vi "StimFile (G3)-Create.vi"(0 "File":T1, 7 "Npts":i32=-1, 11 "error in (no error)":errorcluster) -> (4 "File out":T1, 8 "Y":dbl[](array[numeric]), 15 "error out":errorcluster)   [LabVIEW 2020]
uses:
  Waveform VIs/File VIs/StimFile-Params.ctl
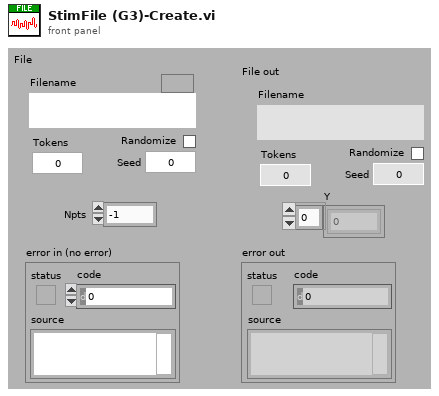
[diagram p1: front panel]
types:
  T1 = typedef "StimFile-Params.ctl" = cluster{"Filename":path, "Signal":dbl[], "Channel":i32, "stream":bool, "offset":i32, "nreps":i32, "loops":i32, "Randomize":bool, "order":i32[], "Seed":i32, "Tokens":i32}
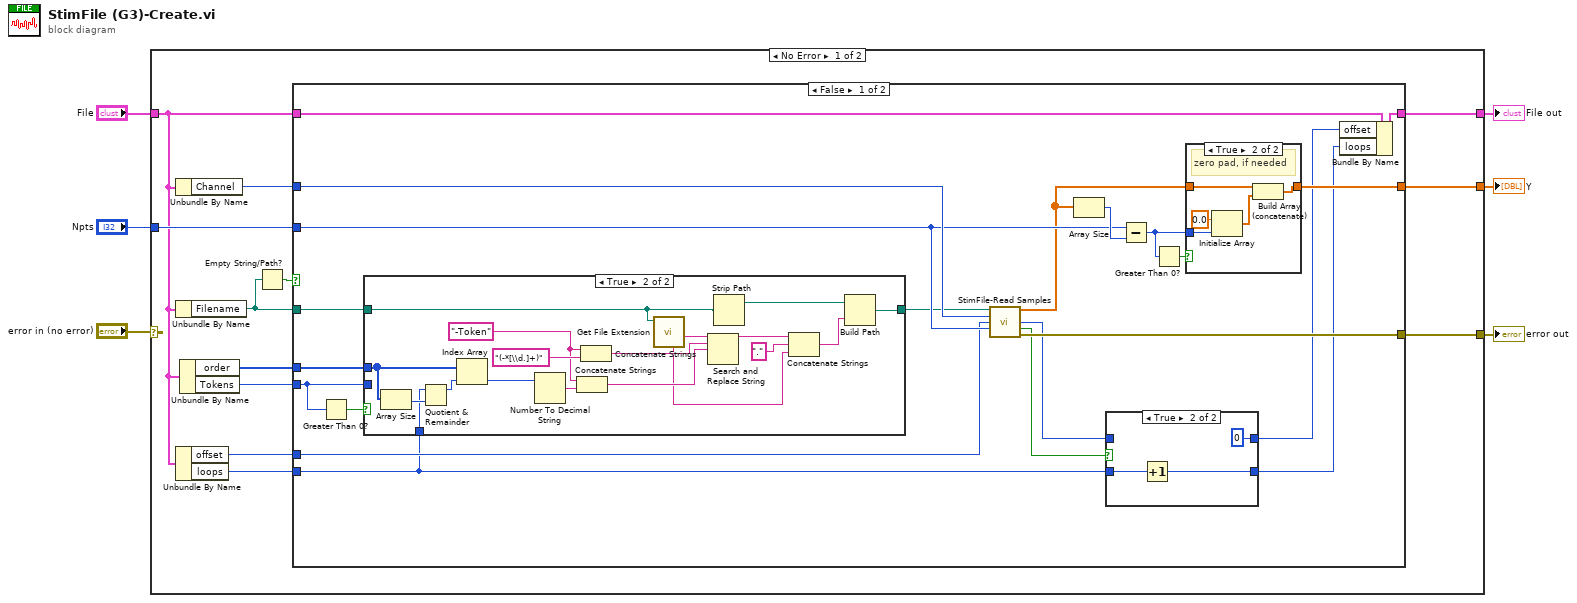
[diagram p0: block diagram]
diagram:
  n1 = case shown="No Error" "error in (no error)" {
    selector: "error in (no error)" -> [_ w71]
    tunnel: "File" -> [w9 _]
    tunnel: "Npts" -> [w17 _]
    tunnel: [w18 w71] -> w3
    tunnel: [w12 _] -> w2
    tunnel: [w11 _] -> w1
    frame No Error {
      n2 = Unbundle By Name(w9) -> ("Channel"=w14:i32)
      n3 = Unbundle By Name(w9) -> ("Filename"=w15:path)
      n4 = Unbundle By Name(w9) -> ("offset"=w13:i32, "loops"=w10:i32)
      n5 = Unbundle By Name(w9) -> ("order"=w7:i32[], "Tokens"=w8:i32)
      n6 = Empty String/Path?(string/path=w15) -> (empty?=w16:bool)
      n7 = case shown="False" w16 {
        tunnel: w15 -> [w24 _]
        tunnel: [w39 _] -> w18
        tunnel: w17 -> [w31 _]
        tunnel: w14 -> [w32 _]
        tunnel: w13 -> [w25 _]
        tunnel: w9 -> [w35 w70]
        tunnel: [w34 w70] -> w12
        tunnel: [w33 _] -> w11
        tunnel: w10 -> [w19 _]
        tunnel: w8 -> [w22 _]
        tunnel: w7 -> [w20 _]
        frame False {
          n8 = Greater Than 0?(x=w22) -> (x > 0?=w23:bool)
          n9 = case shown="True" w23 {
            tunnel: w24 -> [w40 w50]
            tunnel: w22 -> [_ _]
            tunnel: [w40 w48] -> w21
            tunnel: w20 -> [_ w44]
            tunnel: w19 -> [_ w42]
            frame False {
            }
            frame True {
              w57 = "-Token"
              n10 = Array Size(array=w44) -> (size(s)=w43:i32)
              n11 = Quotient & Remainder(x=w42, y=w43) -> (x-y*floor(x/y)=w41:i32)  [unwired: 1 out]
              n12 = Index Array(array=w44, index=w41) -> (element=w56:i32)
              n13 = Number To Decimal String(number=w56) -> (decimal integer string=w55:string)  [unwired: 1 in]
              n14 = Concatenate Strings(w57, w55) -> (w52:string)
              n15 = Concatenate Strings(w57, "(-*[\\d.]+)" ("string")) -> (w53:string)
              n16 = call <vilib>:"Get File Extension.vi"("file"=w50) -> ("filename without extension"=w54:string, "unmodified file extension"=w45:string)  [unwired: 6 in, 3 out]
              n17 = Search and Replace String(input string=w54, search string=w53, replace string=w52) -> (result string=w47:string)  [unwired: 5 in, 3 out]
              n18 = Strip Path(path=w50) -> (stripped path=w49:path)  [unwired: 1 out]
              n19 = Concatenate Strings(w47, "." ("string"), w45) -> (w51:string)
              n20 = Build Path(base path=w49, name or relative path=w51) -> (appended path=w48:path)
            }
          }
          n21 = call "StimFile-Read Samples.vi"("Filename"=w21, "channel"=w32, "offset in"=w25, "Npts"=w31) -> ("Samples"=w30:dbl[], "offset out"=w28:i32, "end of file?"=w29:bool, "error out"=w39:errorcluster)  [unwired: 8 in]
          n22 = Array Size(array=w30) -> (size(s)=w38:i32)
          n23 = case shown="True" w29 {
            tunnel: w19 -> [w60 w62]
            tunnel: w28 -> [w59 _]
            tunnel: [w59 0] -> w27
            tunnel: [w60 w61] -> w26
            frame False {
            }
            frame True {
              n24 = Increment(x=w62) -> (x+1=w61:i32)
            }
          }
          n25 = Subtract(x=w31, y=w38) -> (x-y=w36:i32)
          n26 = Greater Than 0?(x=w36) -> (x > 0?=w37:bool)
          n27 = case shown="True" w37 {
            tunnel: w30 -> [w64 w69]
            tunnel: w36 -> [_ w66]
            tunnel: [w64 w68] -> w33
            frame False {
            }
            frame True {
              # "zero pad, if needed"
              n28 = Initialize Array(0.0 ("element"), w66) -> (w67:dbl[])
              n29 = Build Array (concatenate)(w69, w67) -> (w68:dbl[])
            }
          }
          n30 = Bundle By Name(cluster=w35, "offset"=w27, "loops"=w26) -> (w34:T1)
        }
        frame True {
        }
      }
    }
    frame Error {
    }
  }
  "error out" <- w3
  "File out" <- w2
  "Y" <- w1
